vi "Read Cycle Time (ms).vi"(8 "error in (no error)":errorcluster, 11 "No Query in":refnum<class "No Query.lvclass">) -> (0 "error out":errorcluster, 2 "Cycle Time (ms)":u32, 3 "No Query out":refnum<class "No Query.lvclass">)   [LabVIEW 2018]
doc: "No Query.lvclass:Read Cycle Time (ms).vi\n\nThis VI reads the No Query Class value of the Cycle Time (ms) parameter.\n \nDecember, 2017 Original Code Consulting David Thomson\n www.originalcode.com"
uses:
  No Query.lvclass
  C:/MICAS-X/Drivers/MICM/ICM/Query/Query.lvclass
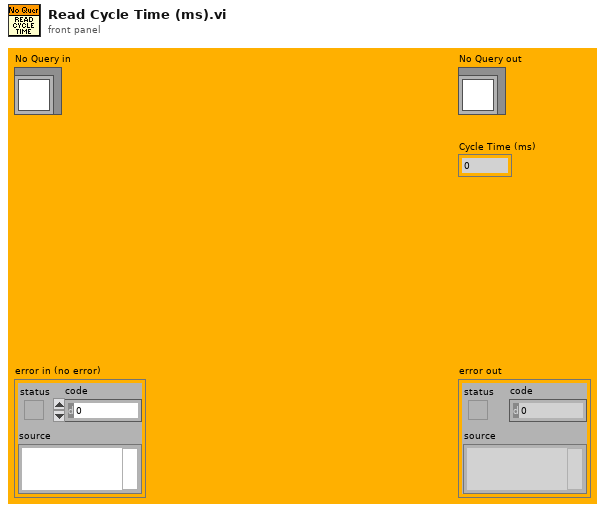
[diagram p1: front panel]
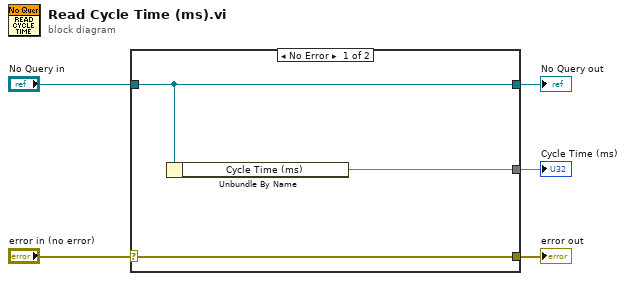
[diagram p0: block diagram]
diagram:
  n1 = case shown="No Error" "error in (no error)" {
    selector: "error in (no error)" -> [w8 w9]
    tunnel: [w8 w9] -> w4
    tunnel: [w7 w10] -> w2
    tunnel: "No Query in" -> [w7 w10]
    tunnel: [w6 _] -> w1
    frame No Error {
      n2 = Unbundle By Name(w7) -> ("Cycle Time (ms)"=w6)
    }
    frame Error {
    }
  }
  "error out" <- w4
  "No Query out" <- w2
  "Cycle Time (ms)" <- w1
